vi "convert_to_photons.vi"(5 "sync_period_ps":i64, 7 "sync_channel":i32, 8 "error in":errorcluster, 10 "data_path":path, 11 "raw_log_path":path) -> (0 "error out":errorcluster)   [LabVIEW 2018]
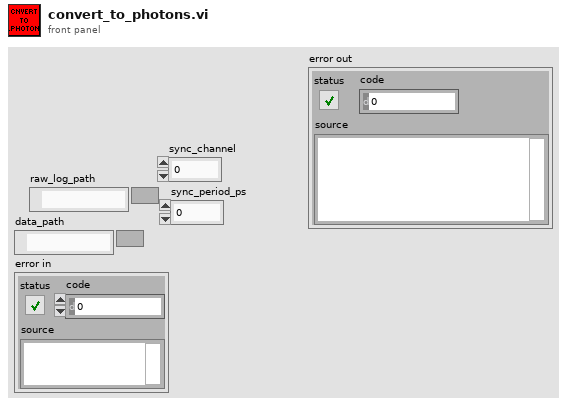
[diagram p1: front panel]
types:
  T1 = enum16{"big-endian, network order", "native, host order", "little-endian"}
  T2 = enum16{"open", "replace", "create", "open or create", "replace or create", "replace or create with confirmation"}
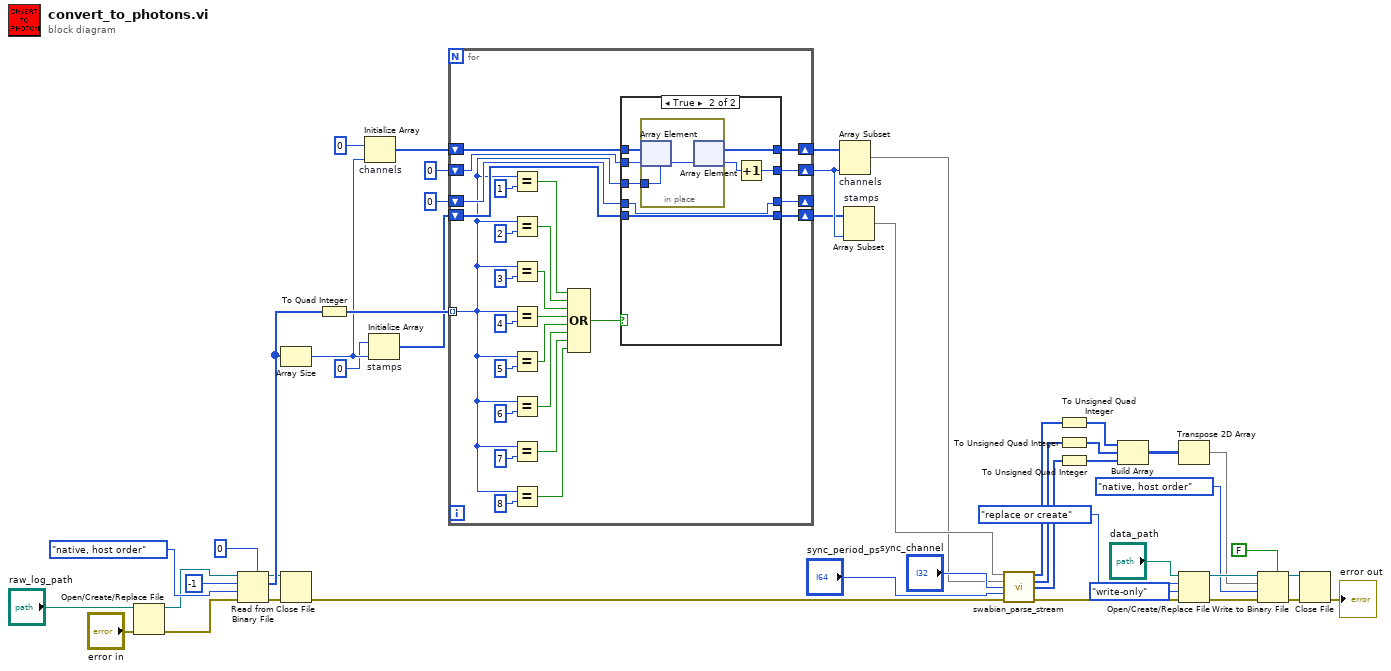
[diagram p0: block diagram]
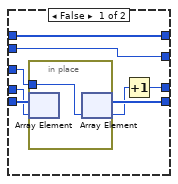
[diagram p2: hidden frame]
diagram:
  n1 = Open/Create/Replace File(file path (use dialog)="raw_log_path", error in="error in") -> (refnum out=w26:refnum<file>, error out=w27:errorcluster)  [unwired: 4 in, 1 out]
  n2 = Read from Binary File(5:u64 0 ("element"), 8:w27, 9:T1."native, host order" ("byte order (0:big-endian, network order)"), 10:-1 ("count (1)"), 11:w26) -> (0:w30:errorcluster, 2:w44:u64[], 3:w29:refnum<file>)  [unwired: 1 in, 1 out]
  n3 = Array Size(array=w44) -> (size(s)=w35:i32)
  n4 = Close File(refnum=w29, error in=w30) -> (error out=w25:errorcluster)  [unwired: 1 out]
  n5 = To Quad Integer(1:w44) -> (0:w40:i64[])
  n6 = Initialize Array "channels"(u32 0 ("element"), w35) -> (w36:u32[])
  n7 = Initialize Array "stamps"(i64 0 ("element"), w35) -> (w38:i64[])
  n8 = for {
    tunnel: w40 -> [w51] mode=indexing
    shift-right: [w67] -> w41
    shift-left: w36 -> [w68]
    shift-right: [w66] -> w43
    shift-left: 0 ("element") -> [w69]
    shift-right: [w64] -> w42
    shift-left: w38 -> [w65]
    shift-right: [w62] -> _
    shift-left: 0 ("element") -> [w63]
    n9 = Equal?(x=w51, y=i64 1) -> (x = y?=w60:bool)
    n10 = Equal?(x=w51, y=i64 2) -> (x = y?=w59:bool)
    n11 = Equal?(x=w51, y=i64 3) -> (x = y?=w57:bool)
    n12 = Equal?(x=w51, y=i64 4) -> (x = y?=w50:bool)
    n13 = Equal?(x=w51, y=i64 5) -> (x = y?=w49:bool)
    n14 = Equal?(x=w51, y=i64 6) -> (x = y?=w48:bool)
    n15 = Equal?(x=w51, y=i64 7) -> (x = y?=w47:bool)
    n16 = Equal?(x=w51, y=i64 8) -> (x = y?=w46:bool)
    n17 = Compound Arithmetic op=OR(w60, w59, w57, w50, w49, w48, w47, w46) -> (w58:bool)
    n18 = case shown="True" w58 {
      tunnel: w69 -> [w79 w85]
      tunnel: w68 -> [w78 w88]
      tunnel: w51 -> [w72 w87]
      tunnel: [w78 w86] -> w67
      tunnel: [w79 w83] -> w66
      tunnel: w65 -> [w77 w81]
      tunnel: [w76 w81] -> w64
      tunnel: w63 -> [w75 w82]
      tunnel: [w73 w82] -> w62
      frame False {
        n19 = in-place {
          in-place-border: w72 -> [w80]
          n20 = in-place-array #1(w77, w75) -> ()  [unwired: 1 out]
          n21 = in-place-array #1(w80) -> (w76:i64[], w74:i32)
        }
        n22 = Increment(x=w74) -> (x+1=w73:i32)
      }
      frame True {
        n23 = in-place {
          in-place-border: w87 -> [w89]
          n24 = in-place-array #2(w88, w85) -> ()  [unwired: 1 out]
          n25 = in-place-array #2(w89) -> (w86:u32[], w84:i32)
        }
        n26 = Increment(x=w84) -> (x+1=w83:i32)
      }
    }
  }
  n27 = Array Subset "channels"(array=w41, length=w43) -> (w1:u32[])  [unwired: 1 in]
  n28 = Array Subset "stamps"(array=w42, length=w43) -> (w2:i64[])  [unwired: 1 in]
  n29 = call "swabian_parse_stream.vi"("stamps"=w2, "channels"=w1, "sync_channel"="sync_channel", "sync_period_ps"="sync_period_ps", "error in (no error)"=w25) -> ("channels"=w22:i32[], "n_sync"=w21:i32[], "delays"=w20:i64[], "error out"=w14:errorcluster)  [unwired: 7 in]
  n30 = To Unsigned Quad Integer(1:w22) -> (0:w19:u64[])
  n31 = To Unsigned Quad Integer(1:w21) -> (0:w18:u64[])
  n32 = To Unsigned Quad Integer(1:w20) -> (0:w17:u64[])
  n33 = Build Array(w19, w18, w17) -> (w16:u64[][])
  n34 = Transpose 2D Array(2D array=w16) -> (transposed array=w11:u64[][])
  n35 = Open/Create/Replace File(file path (use dialog)="data_path", error in=w14, operation (0:open)=T2."replace or create", access (0:read/write)=enum16{"read/write", "read-only", "write-only"}."write-only") -> (refnum out=w12:refnum<file>, error out=w13:errorcluster)  [unwired: 2 in, 1 out]
  n36 = Write to Binary File(file (use dialog)=w12, data=w11, error in=w13, 5:FALSE ("prepend array or string size? (T)"), 9:T1."native, host order" ("byte order (0:big-endian, network order)")) -> (refnum out=w7:refnum<file>, error out=w8:errorcluster)  [unwired: 1 in, 1 out]
  n37 = Close File(refnum=w7, error in=w8) -> (error out=→"error out":errorcluster)  [unwired: 1 out]
